vi "violet--constant.vi"() -> (1 "Violet":u32(colorbox))   [LabVIEW 2018]
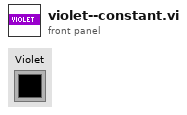
[diagram p1: front panel]
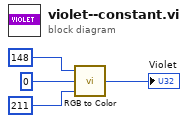
[diagram p0: block diagram]
diagram:
  n1 = call <vilib>:"RGB to Color.vi"("B"=u8 211, "G"=u8 0, "R"=u8 148) -> ("Color"=→"Violet":u32)
